vi "Tell.vi"(4 "Priority":bool, 10 "Msg":refnum<class "Msg.lvclass">, 11 "Queue Transport in":refnum<class "Queue Transport.lvclass">) -> (0 "Error out":errorcluster)   [LabVIEW 2025, in "jettl.lvlib" / "Transport.lvlib" / "Queue.lvlib" / "Queue Transport.lvclass"]
uses:
  Queue Transport.lvclass
  Msg/Msg.lvclass
  Queue Transport.lvclass/Queue Transport.ctl
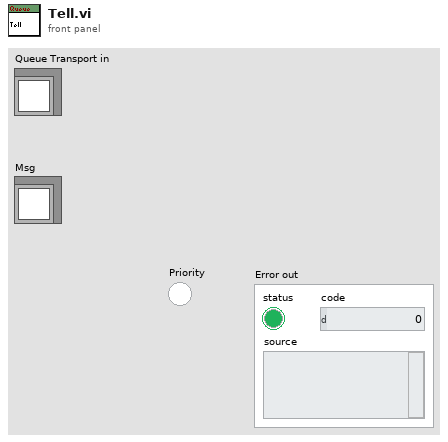
[diagram p1: front panel]
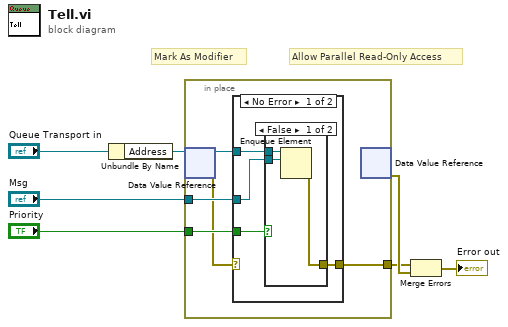
[diagram p0: block diagram]
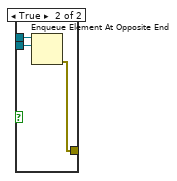
[diagram p2: hidden frame]
diagram:
  # "Allow Parallel Read-Only Access"
  # "Mark As Modifier"
  n1 = Unbundle By Name("Queue Transport in") -> ("Address"=w4:refnum<data-value>)
  n2 = in-place {
    in-place-border: [w12] -> w1
    in-place-border: "Msg" -> [w11]
    in-place-border: "Priority" -> [w10]
    n3 = in-place-dvr #1(w4) -> (w9:refnum<queue>, w8:errorcluster)
    n4 = case shown="No Error" w8 {
      selector: w8 -> [_ w23]
      tunnel: [w16 w23] -> w12
      tunnel: w11 -> [w15 _]
      tunnel: w10 -> [w14 _]
      tunnel: w9 -> [w13 _]
      frame No Error {
        n5 = case shown="False" w14 {
          tunnel: w13 -> [w19 w22]
          tunnel: [w18 w20] -> w16
          tunnel: w15 -> [w17 w21]
          frame False {
            n6 = Enqueue Element(queue=w19, element=w17) -> (error out=w18:errorcluster)  [unwired: 2 in, 2 out]
          }
          frame True {
            n7 = Enqueue Element At Opposite End(queue=w22, element=w21) -> (error out=w20:errorcluster)  [unwired: 2 in, 2 out]
          }
        }
      }
      frame Error {
      }
    }
    n8 = in-place-dvr #1() -> (w2:errorcluster)  [unwired: 1 in, 1 out]
  }
  n9 = Merge Errors(w1, w2) -> (→"Error out":errorcluster)
